vi "Delete Tree Priv.vi"(8 "Error In":errorcluster, 10 "Unique ID":string, 11 "Tree Dictionary In":variant) -> (0 "Error Out":errorcluster, 3 "Tree Dictionary Out":variant)   [LabVIEW 2017, in "Tree API.lvlib" / "Tree.lvclass"]
uses:
  Tree.lvclass
  Typedefs/Tree Cluster.ctl
  Tree Data/Tree Data.lvclass
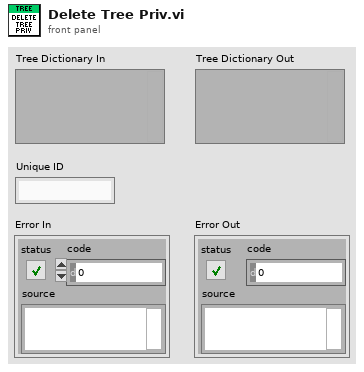
[diagram p1: front panel]
types:
  T1 = typedef "Tree API.lvlib/Tree.lvclass/Tree Cluster.ctl" = cluster{"Unique ID":string, "Parent ID":string, "Child IDs":string[], "Name":string, "MetaData":string, "Data IDs":string[]}
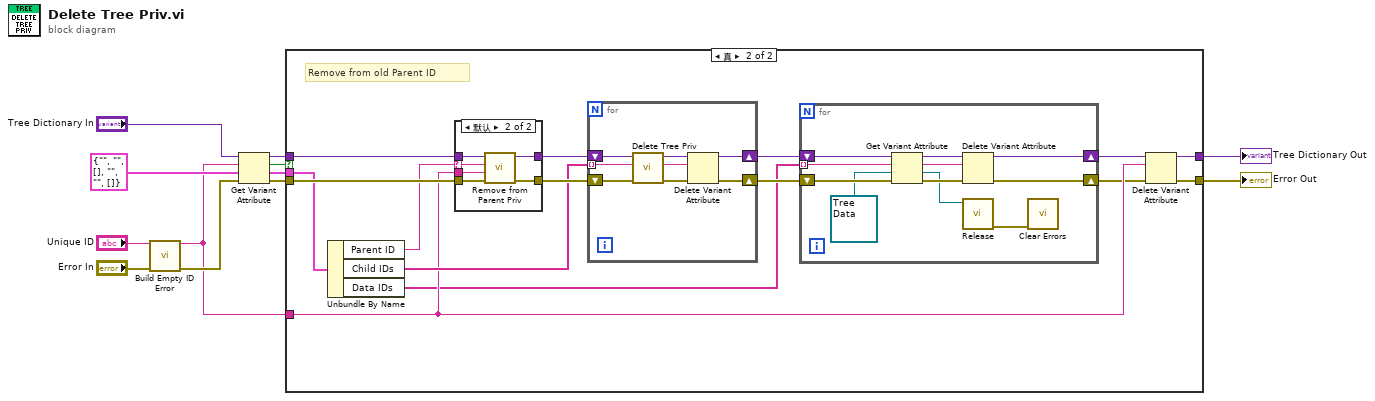
[diagram p0: block diagram]
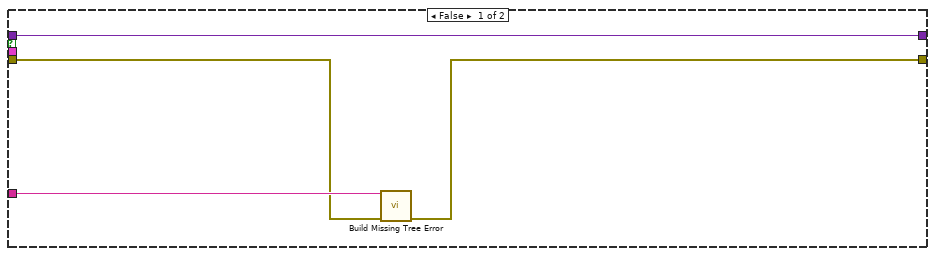
[diagram p2: hidden frame]
diagram:
  n1 = call "Build Empty ID Error.vi"("Unique ID"="Unique ID", "Error In"="Error In") -> ("Unique ID Out"=w1:string, "Error Out"=w2:errorcluster)  [unwired: 12 in]
  n2 = Get Variant Attribute(Variant="Tree Dictionary In", name=w1, default value (empty Variant)=T1 {"Unique ID"="", "Parent ID"="", "Child IDs"=[], "Name"="", "MetaData"="", "Data IDs"=[]} ("Cluster of class private data"), error in=w2) -> (duplicate Variant=w7:variant, found=w9:bool, value=w8:T1, error out=w6:errorcluster)
  n3 = case shown="真" w9 {
    tunnel: w8 -> [_ w30]
    tunnel: w7 -> [w16 w29]
    tunnel: w6 -> [w13 w31]
    tunnel: [w14 w25] -> w11
    tunnel: [w16 w24] -> w12
    tunnel: w1 -> [w15 w23]
    frame False {
      n4 = call "Build Missing Tree Error.vi"("Unique ID"=w15, "Error In"=w13) -> ("Error Out"=w14:errorcluster)  [unwired: 13 in]
    }
    frame True {
      # "Remove from old Parent ID"
      n5 = Unbundle By Name(w30) -> ("Parent ID"=w22:string, "Child IDs"=w26:string[], "Data IDs"=w17:string[])
      n6 = case shown="默认" w22 {
        selector: w22 -> [_ w44]
        tunnel: w31 -> [w42 w49]
        tunnel: w29 -> [w43 w48]
        tunnel: [w43 w47] -> w28
        tunnel: [w42 w46] -> w27
        tunnel: w23 -> [_ w45]
        frame "" {
        }
        frame Default {
          n7 = call "Remove from Parent Priv.vi"("Error In"=w49, "Unique ID"=w45, "Parent ID"=w44, "Tree Dictionary"=w48) -> ("Error Out"=w46:errorcluster, "Tree Dictionary Out"=w47:variant)  [unwired: 6 in]
        }
      }
      n8 = for {
        shift-right: [w51] -> w18
        shift-left: w27 -> [w55]
        shift-right: [w50] -> w21
        shift-left: w28 -> [w56]
        tunnel: w26 -> [w52] mode=indexing
        n9 = call "Delete Tree Priv.vi"("Error In"=w55, "Unique ID"=w52, "Tree Dictionary In"=w56) -> ("Error Out"=w53:errorcluster, "Tree Dictionary Out"=w54:variant)  [unwired: 7 in]
        n10 = Delete Variant Attribute(4:w53, 6:w52, 7:w54) -> (0:w51:errorcluster, 3:w50:variant)  [unwired: 1 out]
      }
      n11 = for {
        shift-right: [w34] -> w20
        shift-left: w21 -> [w41]
        shift-right: [w33] -> w19
        shift-left: w18 -> [w40]
        tunnel: w17 -> [w37] mode=indexing
        n12 = Get Variant Attribute(Variant=w41, name=w37, default value (empty Variant)=refnum<class "Tree Data.lvclass"> refnum ("Tree API.lvlib:Tree Data.lvclass"), error in=w40) -> (duplicate Variant=w39:variant, value=w35:refnum<class "Tree Data.lvclass">, error out=w36:errorcluster)  [unwired: 1 out]
        n13 = Delete Variant Attribute(4:w36, 6:w37, 7:w39) -> (0:w33:errorcluster, 3:w34:variant)  [unwired: 1 out]
        n14 = call-dynamic "Release.vi"("Tree Data"=w35) -> ("Error Out"=w32:errorcluster)  [unwired: 10 in]
        n15 = call <vilib>:"Clear Errors.vi"("error in (no error)"=w32) -> ()  [unwired: 5 in, 2 out]
      }
      n16 = Delete Variant Attribute(4:w19, 6:w23, 7:w20) -> (0:w25:errorcluster, 3:w24:variant)  [unwired: 1 out]
    }
  }
  "Tree Dictionary Out" <- w12
  "Error Out" <- w11
